vi "AtlasDisconnect.vi"(8 "error in (no error)":errorcluster) -> (0 "error out":errorcluster)   [LabVIEW 2017]
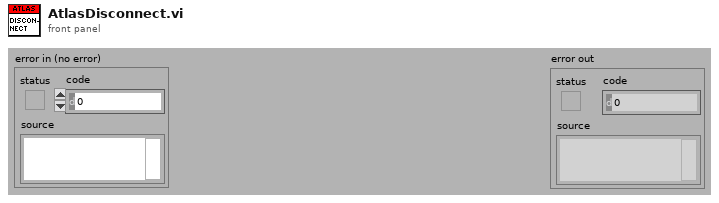
[diagram p1: front panel]
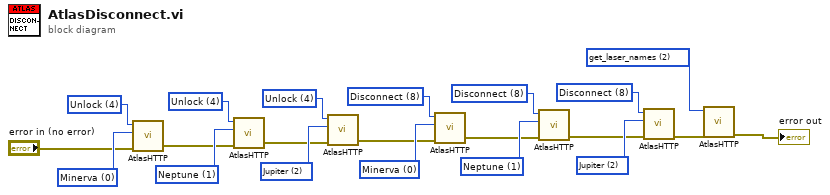
[diagram p0: block diagram]
diagram:
  w9 = u16 2 items=["Login", "Logout", "get_laser_names", "Ping", "Unlock", "Lock171", "Lock174", "Connect", "Disconnect"] ("Command")
  w10 = u16 2 items=["Minerva", "Neptune", "Jupiter"] ("Laser")
  w11 = u16 8 items=["Login", "Logout", "get_laser_names", "Ping", "Unlock", "Lock171", "Lock174", "Connect", "Disconnect"] ("Command")
  w12 = u16 1 items=["Minerva", "Neptune", "Jupiter"] ("Laser")
  w13 = u16 8 items=["Login", "Logout", "get_laser_names", "Ping", "Unlock", "Lock171", "Lock174", "Connect", "Disconnect"] ("Command")
  w14 = u16 0 items=["Minerva", "Neptune", "Jupiter"] ("Laser")
  w15 = u16 8 items=["Login", "Logout", "get_laser_names", "Ping", "Unlock", "Lock171", "Lock174", "Connect", "Disconnect"] ("Command")
  w16 = u16 2 items=["Minerva", "Neptune", "Jupiter"] ("Laser")
  w17 = u16 4 items=["Login", "Logout", "get_laser_names", "Ping", "Unlock", "Lock171", "Lock174", "Connect", "Disconnect"] ("Command")
  w18 = u16 1 items=["Minerva", "Neptune", "Jupiter"] ("Laser")
  w19 = u16 4 items=["Login", "Logout", "get_laser_names", "Ping", "Unlock", "Lock171", "Lock174", "Connect", "Disconnect"] ("Command")
  w20 = u16 0 items=["Minerva", "Neptune", "Jupiter"] ("Laser")
  w21 = u16 4 items=["Login", "Logout", "get_laser_names", "Ping", "Unlock", "Lock171", "Lock174", "Connect", "Disconnect"] ("Command")
  n1 = call "AtlasHTTP.vi"("error in (no error)"="error in (no error)", "Laser"=w20, "Command"=w21) -> ("error out"=w3:errorcluster)  [unwired: 5 in, 1 out]
  n2 = call "AtlasHTTP.vi"("error in (no error)"=w3, "Laser"=w18, "Command"=w19) -> ("error out"=w4:errorcluster)  [unwired: 5 in, 1 out]
  n3 = call "AtlasHTTP.vi"("error in (no error)"=w4, "Laser"=w16, "Command"=w17) -> ("error out"=w5:errorcluster)  [unwired: 5 in, 1 out]
  n4 = call "AtlasHTTP.vi"("error in (no error)"=w5, "Laser"=w14, "Command"=w15) -> ("error out"=w6:errorcluster)  [unwired: 5 in, 1 out]
  n5 = call "AtlasHTTP.vi"("error in (no error)"=w6, "Laser"=w12, "Command"=w13) -> ("error out"=w7:errorcluster)  [unwired: 5 in, 1 out]
  n6 = call "AtlasHTTP.vi"("error in (no error)"=w7, "Laser"=w10, "Command"=w11) -> ("error out"=w8:errorcluster)  [unwired: 5 in, 1 out]
  n7 = call "AtlasHTTP.vi"("error in (no error)"=w8, "Command"=w9) -> ("error out"=→"error out":errorcluster)  [unwired: 6 in, 1 out]
